vi "SaveCluster (SubVI).vi"(1 "selected path":path, 2 "Datenspeicher 2":refnum<vi>) -> (0 "Kein Fehler":bool)   [LabVIEW 2014]
uses:
  <vilib>/Utility/xml.llb/Write to XML File(string).vi
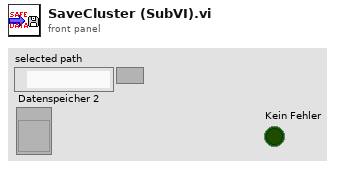
[diagram p1: front panel]
types:
  T1 = cluster{"Fahrzeugdaten":string, "date/time string":string, "Rolle [Inkr/U]":u16, "Rollenumfang [m]":dbl, "Rollenträgheit [kgm²]":dbl, "Zündung [Imp/U]":dbl, "Getriebe [1:]":dbl, "Reifenumfang [m] ":dbl, "element":dbl, "Gl. Mittelwert":u8, "Differenzenquotient":u8, "Polynom":u8, "dT [s]":dbl, "element":dbl, "Lufttemperatur [°C]":dbl, "Luftfeuchtigkeit [%]":dbl, "Luftdruck [mbar]":dbl, dbl[], dbl[], "Best Polynomial Fit":dbl[], dbl[], "Übersetzung ermitteln aus":u8, "[s]":dbl, "nmin [1/min]":dbl, "nmax [1/min]":dbl, "n vom Gas [1/min]":dbl, "dT ungefiltert [s]":dbl[], i32[], "Boolesch":bool, "Serielle Schnittstelle":refnum<visa-resource-name>, "nKuWe/nRolle 2":dbl, "v vom Gas [km/h]":dbl}
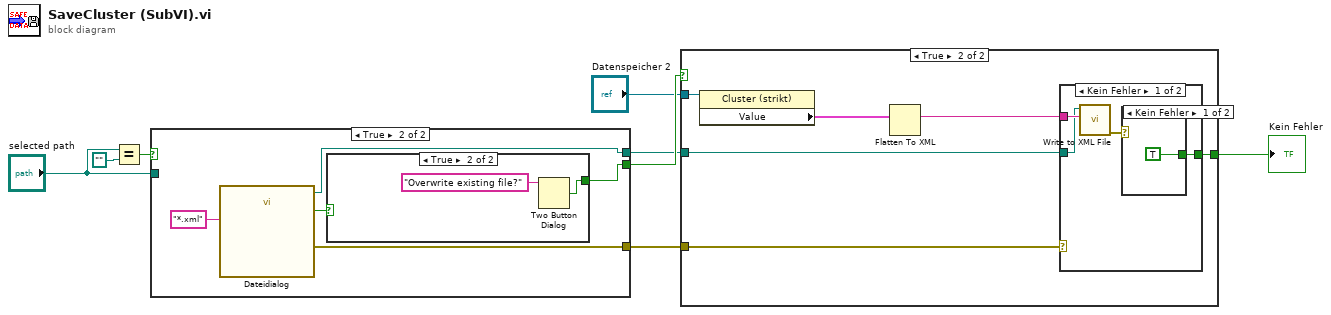
[diagram p0: block diagram]
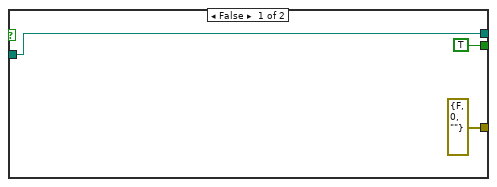
[diagram p2: hidden frame]
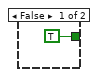
[diagram p3: hidden frame]
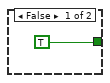
[diagram p4: hidden frame]
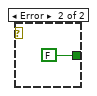
[diagram p5: hidden frame]
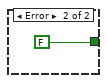
[diagram p6: hidden frame]
diagram:
  n1 = Equal?(x="selected path", y=path "") -> (x = y?=w5:bool)
  n2 = case shown="True" w5 {
    tunnel: [TRUE ("T button?") w16] -> w8
    tunnel: [errorcluster {"status"=FALSE, "code"=0, "source"=""} ("error out") w14] -> w7
    tunnel: [w10 w13] -> w6
    tunnel: "selected path" -> [w10 _]
    frame False {
    }
    frame True {
      n3 = call "Dateidialog"("pattern (all files)"="*.xml") -> ("selected path"=w13:path, "exists"=w15:bool, "error out"=w14:errorcluster)  [unwired: 11 in, 1 out]
      n4 = case shown="True" w15 {
        tunnel: [TRUE ("T button?") w18] -> w16
        frame False {
        }
        frame True {
          n5 = Two Button Dialog(message="Overwrite existing file?" ("Nachricht")) -> (T button?=w18:bool)  [unwired: 2 in]
        }
      }
    }
  }
  n6 = case shown="True" w8 {
    tunnel: w6 -> [_ w26]
    tunnel: w7 -> [_ w25]
    tunnel: "Datenspeicher 2" -> [_ w23]
    tunnel: [TRUE w21] -> w1
    frame False {
    }
    frame True {
      n7 = property class="Cluster (strikt)"(reference=w23) -> ("Value"=w22:T1)  [unwired: 1 in, 2 out]
      n8 = Flatten To XML(anything=w22) -> (xml string=w24:string)
      n9 = case shown="Kein Fehler" w25 {
        tunnel: w24 -> [w30 _]
        tunnel: w26 -> [w28 _]
        tunnel: [w27 FALSE] -> w21
        frame No Error {
          n10 = call-poly <vilib>:"Write to XML File.vi"("XML Input"=w30, "XML File Path"=w28) -> ("error out"=w29:errorcluster)  [unwired: 7 in, 2 out]
          n11 = case shown="Kein Fehler" w29 {
            tunnel: [TRUE FALSE] -> w27
            frame No Error {
            }
            frame Error {
            }
          }
        }
        frame Error {
        }
      }
    }
  }
  "Kein Fehler" <- w1
